vi "Check Valid UI Selection.vi"(8 "error in (no error)":errorcluster, 11 "Operator UI in":refnum<class "Measurement UI.lvclass">) -> (0 "error out":errorcluster, 3 "Operator UI out":refnum<class "Measurement UI.lvclass">)   [LabVIEW 2016, in "Measurement UI.lvlib" / "Measurement UI.lvclass"]
uses:
  Measurement UI.lvclass
  Measurement UI.lvclass/Measurement UI.ctl
  Accessors/Read settings button array for hardware.vi
  Accessors/Read Run.vi
  Read Multimeter.vi
  Accessors/Read Digitizer.vi
  Accessors/Read Function Generator.vi
  Read Run Indefinitely.vi
  Accessors/Read Show FP_.vi
  Accessors/Read Measurement.vi
  Accessors/Read Step Iterations.vi
panel:
  out "Array":string[](array[string])
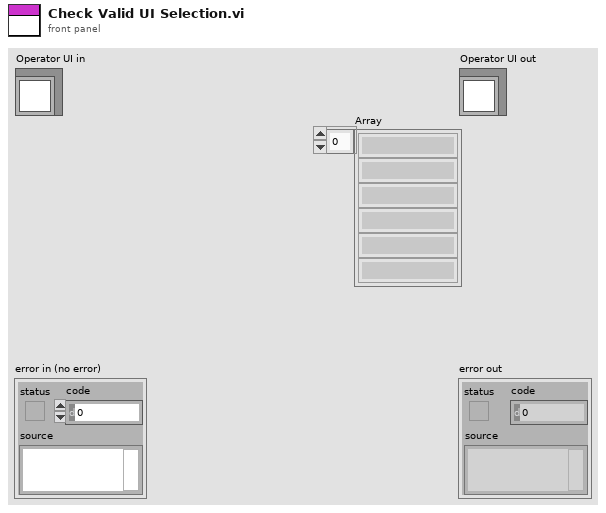
[diagram p1: front panel]
types:
  T1 = enum8{"Enabled", "Disabled", "Disabled and Grayed Out"}
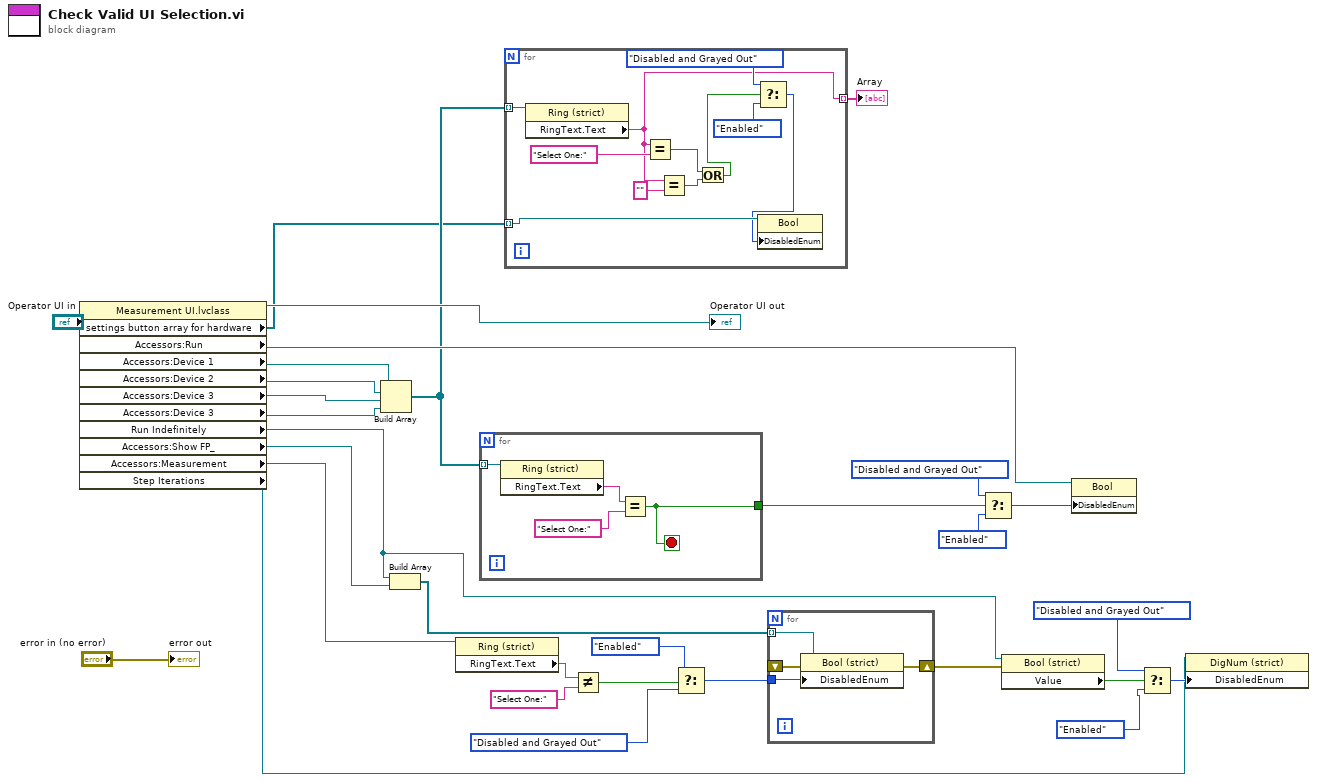
[diagram p0: block diagram]
diagram:
  n1 = property class="Measurement UI.lvclass"(reference="Operator UI in") -> (reference out=→"Operator UI out":refnum<class "Measurement UI.lvclass">, "settings button array for hardware"=w2:refnum<vi>[], "Accessors:Run"=w20:refnum<vi>, "Accessors:Device 1"=w21:refnum<vi>, "Accessors:Device 2"=w22:refnum<vi>, "Accessors:Device 3"=w23:refnum<vi>, "Accessors:Device 3"=w24:refnum<vi>, "Run Indefinitely"=w10:refnum<vi>, "Accessors:Show FP_"=w12:refnum<vi>, "Accessors:Measurement"=w13:refnum<vi>, "Step Iterations"=w5:refnum<vi>)  [unwired: 1 in, 1 out]
  n2 = Build Array(w21, w22, w23, w24) -> (w3:refnum<vi>[])
  n3 = Build Array(w10, w12) -> (w11:refnum<vi>[])
  n4 = property class="Ring (strict)"(reference=w13) -> ("RingText.Text"=w19:string)  [unwired: 1 in, 2 out]
  n5 = for {
    tunnel: w3 -> [w35] mode=indexing
    tunnel: [w32] -> w28
    stop <- w32 stop-if-true
    n6 = property class="Ring (strict)"(reference=w35) -> ("RingText.Text"=w34:string)  [unwired: 1 in, 2 out]
    n7 = Equal?(x=w34, y="Select One:") -> (x = y?=w32:bool)
  }
  n8 = for {
    tunnel: w3 -> [w46] mode=indexing
    tunnel: w2 -> [w45] mode=indexing
    tunnel: [w40] -> w1 mode=indexing
    n9 = property class="Ring (strict)"(reference=w46) -> ("RingText.Text"=w40:string)  [unwired: 1 in, 2 out]
    n10 = Equal?(x=w40, y="Select One:") -> (x = y?=w37:bool)
    n11 = Equal?(x=w40, y="") -> (x = y?=w38:bool)
    n12 = Or(x=w37, y=w38) -> (x .or. y?=w36:bool)
    n13 = Select(t=T1."Disabled and Grayed Out" ("Disabled"), s=w36, f=T1."Enabled" ("Disabled")) -> (s? t:f=w42:T1)
    n14 = property class="Bool"(reference=w45, "DisabledEnum"=w42) -> ()  [unwired: 1 in, 2 out]
  }
  "Array" <- w1
  n15 = Not Equal?(x=w19, y="Select One:") -> (x != y?=w17:bool)
  n16 = Select(t=T1."Enabled" ("Disabled"), s=w17, f=T1."Disabled and Grayed Out" ("Disabled")) -> (s? t:f=w14:T1)
  n17 = for {
    tunnel: w14 -> [w50]
    tunnel: w11 -> [w49] mode=indexing
    shift-right: [w48] -> w4
    shift-left: _ -> [w47]
    n18 = property class="Bool (strict)"(reference=w49, error in=w47, "DisabledEnum"=w50) -> (error out=w48:errorcluster)  [unwired: 1 out]
  }
  n19 = Select(t=T1."Disabled and Grayed Out" ("Disabled"), s=w28, f=T1."Enabled" ("Disabled")) -> (s? t:f=w29:T1)
  n20 = property class="Bool (strict)"(reference=w10, error in=w4) -> ("Value"=w9:bool)  [unwired: 2 out]
  n21 = property class="Bool"(reference=w20, "DisabledEnum"=w29) -> ()  [unwired: 1 in, 2 out]
  n22 = Select(t=T1."Disabled and Grayed Out" ("Disabled"), s=w9, f=T1."Enabled" ("Disabled")) -> (s? t:f=w6:T1)
  n23 = property class="DigNum (strict)"(reference=w5, "DisabledEnum"=w6) -> ()  [unwired: 1 in, 2 out]
  "error out" <- "error in (no error)"
